vi "Calib_Analyse_fit.vi"(0 "Calib file":path, 1 "Input points":dbl[][](array[numeric]) format="%.2f", 2 "polynomial order":i32=2, 5 "Fixed n":bool=TRUE, 7 "n":dbl=0.45 format="%.2f", 9 "Point selector 3":cluster{"Y":dbl, "X":dbl, "t/f":bool}[](array[cluster]) {"X" format="%.2f"; "Y" format="%.2f"}, 11 "Point selector 4":T1(array[cluster])=[{"Y"=3.5155385742, "Y2"=3.2773117676, "X"=-15.0, "t/f"=FALSE}, {"Y"=3.4946367187, "Y2"=3.3075422363, "X"=-10.0, "t/f"=FALSE}, {"Y"=3.473232666, "Y2"=3.3353713379, "X"=-5.0, "t/f"=FALSE}, {"Y"=3.454592041, "Y2"=3.3658986816, "X"=0.0, "t/f"=FALSE}, {"Y"=3.4246572266, "Y2"=3.3874455566, "X"=5.0, "t/f"=FALSE}, {"Y"=3.398965332, "Y2"=3.4137351074, "X"=10.0, "t/f"=FALSE}, {"Y"=3.362712646484375, "Y2"=3.428485595703125, "X"=15.0, "t/f"=FALSE}] {"Y2" format="%.2f"; "X" format="%.2f"; "Y" format="%.2f"}) -> (4 "Calib const":string[][](array[string])=[["n", "0.405000"], ["A", "7.730378"], ["B", "6.204067"], ["Av % err", "0.204301"]], 6 "Calibration plot":cluster{cluster{dbl, dbl}[]}[](graph)=[{[{0.8450215822560672, 12.972948762710196}, {0.9063644870167936, 13.35352428024258}, {1.0129933166229186, 14.015056729178777}, {1.0924501688964157, 14.50801239851709}, {1.2215481063301497, 15.308944707524116}, {1.3521910897315237, 16.119462585897956}, {1.4772434835777744, 16.895296069694275}]}, {[{0.8450215822560672, 12.97084622363197}, {0.9063644870167936, 13.353228276297402}, {1.0129933166229186, 14.026771757587431}, {1.0924501688964157, 14.499243467101884}, {1.2215481063301497, 15.307992219000921}, {1.3521910897315237, 16.116882250583185}, {1.4772434835777744, 16.898281339562185}]}], 8 "Average Temp":dbl=19.0 format="%.2f", 10 "Point selector 3 out":cluster{"Y":dbl, "X":dbl, "t/f":bool}[](array[cluster]) {"X" format="%.2f"; "Y" format="%.2f"}, 14 "Coefficients":dbl[][](array[numeric]) format="%.2f", 15 "Point selector 4 out":T1(array[cluster])=[{"Y"=3.5155385742, "Y2"=3.2773117676, "X"=-15.0, "t/f"=FALSE}, {"Y"=3.4946367187, "Y2"=3.3075422363, "X"=-10.0, "t/f"=FALSE}, {"Y"=3.473232666, "Y2"=3.3353713379, "X"=-5.0, "t/f"=FALSE}, {"Y"=3.454592041, "Y2"=3.3658986816, "X"=0.0, "t/f"=FALSE}, {"Y"=3.4246572266, "Y2"=3.3874455566, "X"=5.0, "t/f"=FALSE}, {"Y"=3.398965332, "Y2"=3.4137351074, "X"=10.0, "t/f"=FALSE}, {"Y"=3.362712646484375, "Y2"=3.428485595703125, "X"=15.0, "t/f"=FALSE}] {"Y2" format="%.2f"; "X" format="%.2f"; "Y" format="%.2f"})   [LabVIEW 2022 SP3]
uses:
  <vilib>/Analysis/baseanly.llb/Mean (DBL).vi
  Globals/Calib_global.vi
  Acquisition/PWA/PWAtasksGLOBAL.vi
  <vilib>/Analysis/NI_AALBase.lvlib
panel:
  out "GMU:Source:ppm/%Density":dbl format="%.2f"
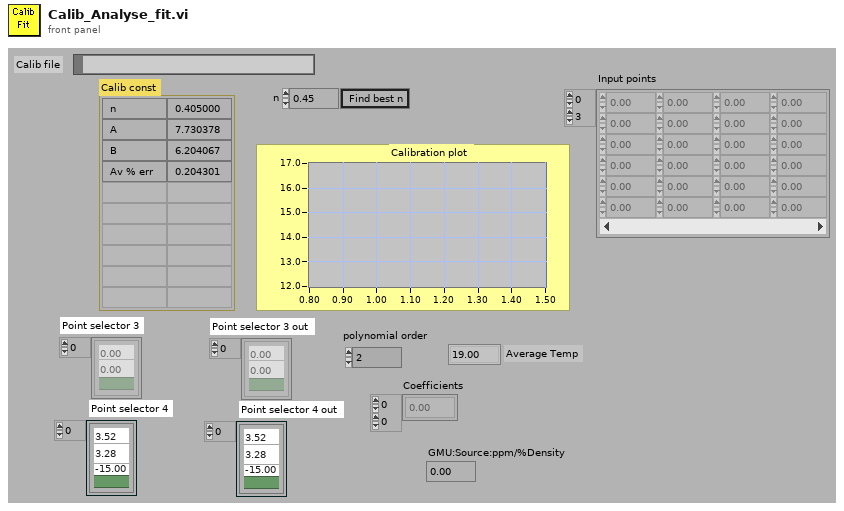
[diagram p1: front panel]
types:
  T1 = cluster{"Y":dbl, "Y2":dbl, "X":dbl, "t/f":bool}[]
  T2 = typedef "Cal_Inst_type.ctl" = enum16{"Propeller anemometer", "Pressure Transducer", "Hot wire", "Cross wire velocity", "Cross wire angle", "Generic Linear", "Generic Polynomial", "Poly Fit Special", "Fast FID", "Thermocouple", "Cold wire", "Pulsed Wire"}
  T3 = cluster{"Y":dbl, "Y":dbl, "X":dbl, "switch":bool}
  T4 = typedef "Ref_Inst_type.ctl" = enum16{"Propellor anemometer", "Pressure Transducer", "Raw voltage", "Pitot-static tube", "Generic Linear", "Generic Polynomial", "Thermocouple", "LDA", "Enter Value", "ADAM Channel"}
  T5 = typedef "zeroableInst.ctl" = enum32{"Zeroable", "Do Not Zero"}
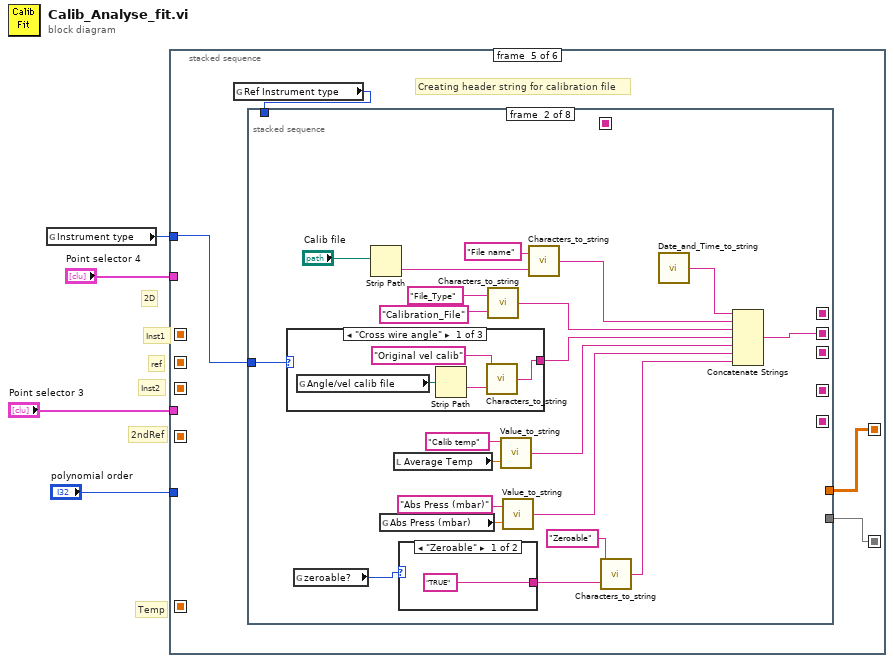
[diagram p0: block diagram]
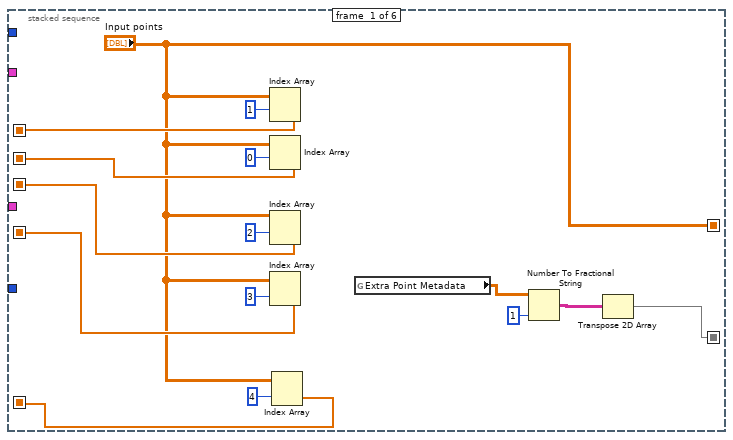
[diagram p2: hidden frame]
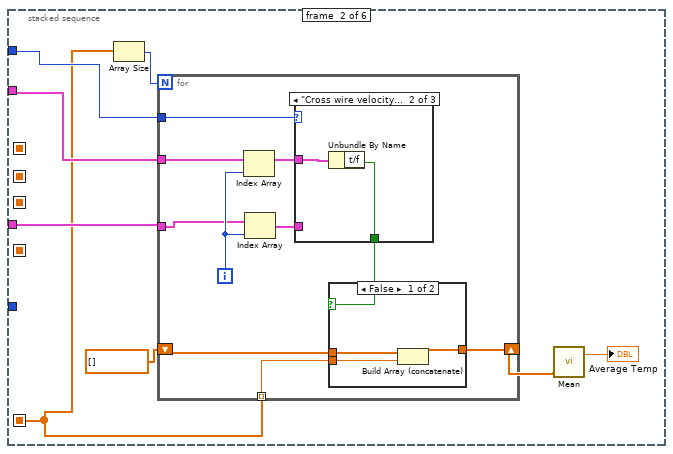
[diagram p3: hidden frame]
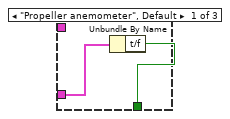
[diagram p5: hidden frame]
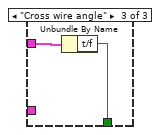
[diagram p6: hidden frame]
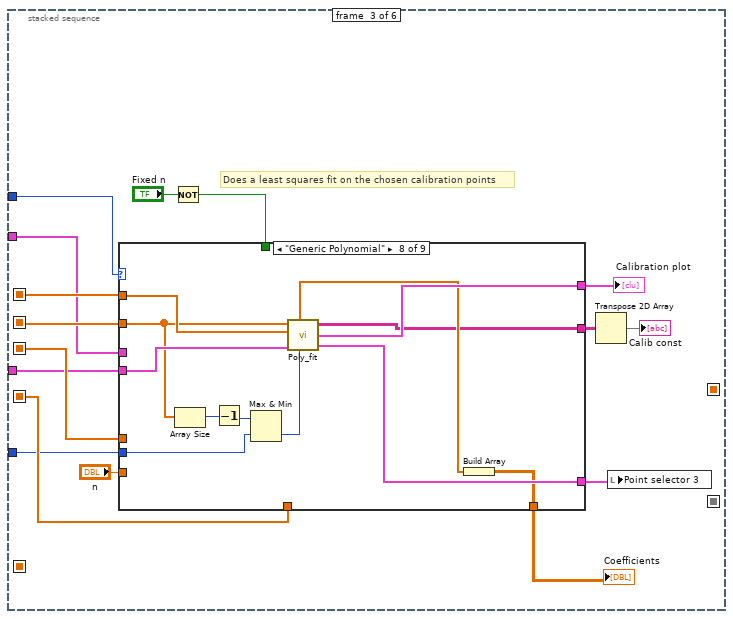
[diagram p7: hidden frame]
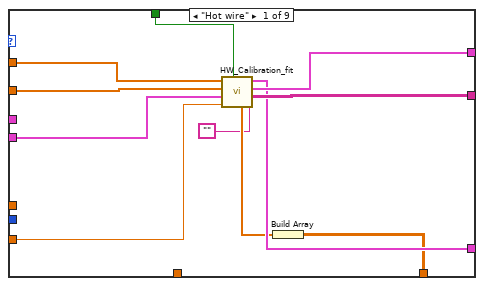
[diagram p8: hidden frame]
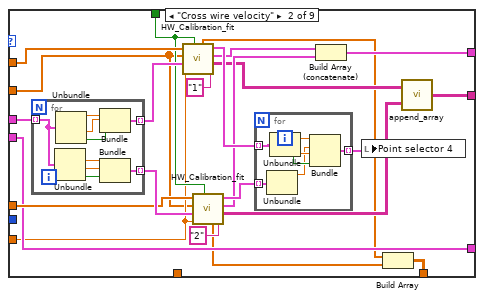
[diagram p9: hidden frame]
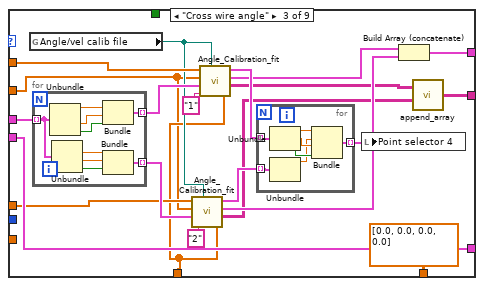
[diagram p10: hidden frame]
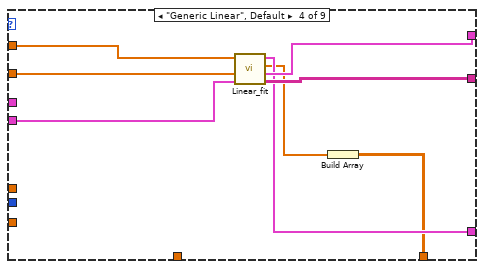
[diagram p11: hidden frame]
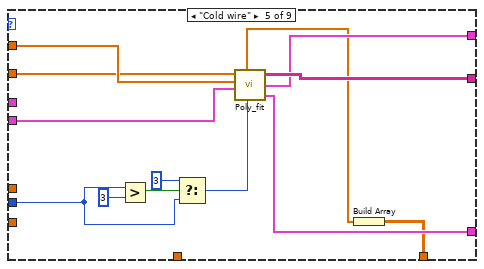
[diagram p12: hidden frame]
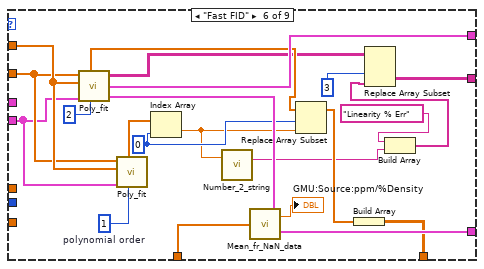
[diagram p13: hidden frame]
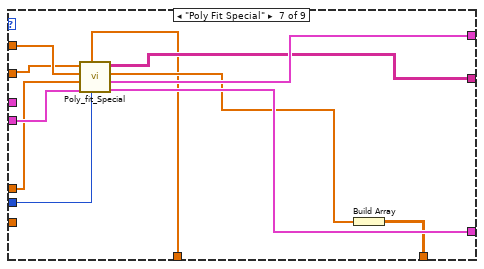
[diagram p14: hidden frame]
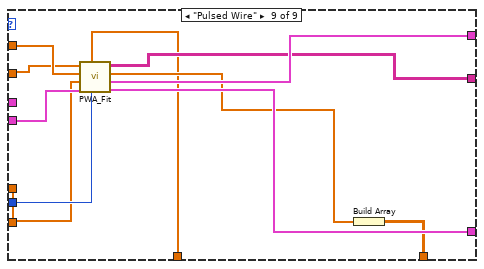
[diagram p15: hidden frame]
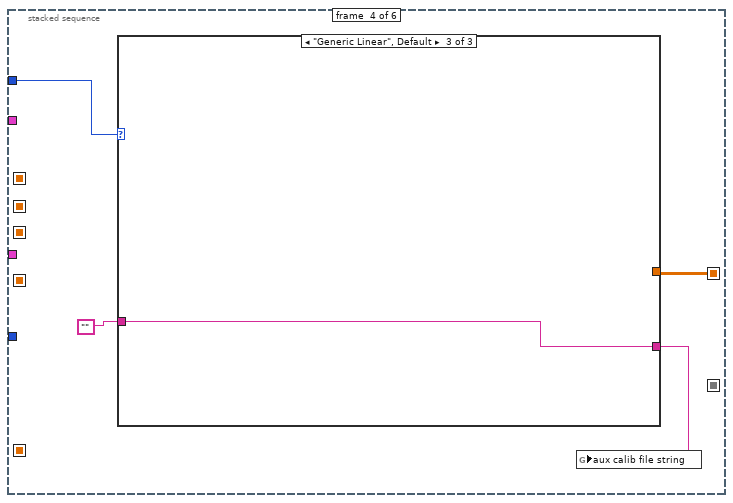
[diagram p16: hidden frame]
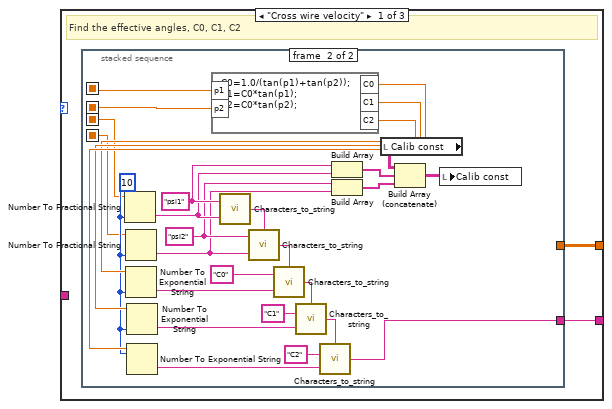
[diagram p17: hidden frame]
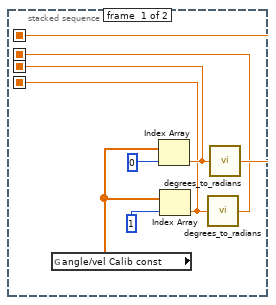
[diagram p18: hidden frame]
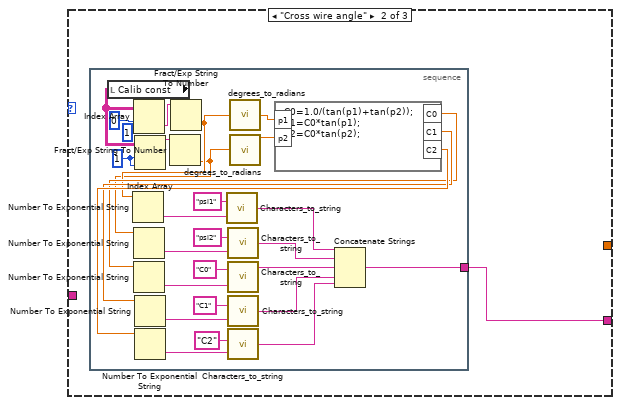
[diagram p19: hidden frame]
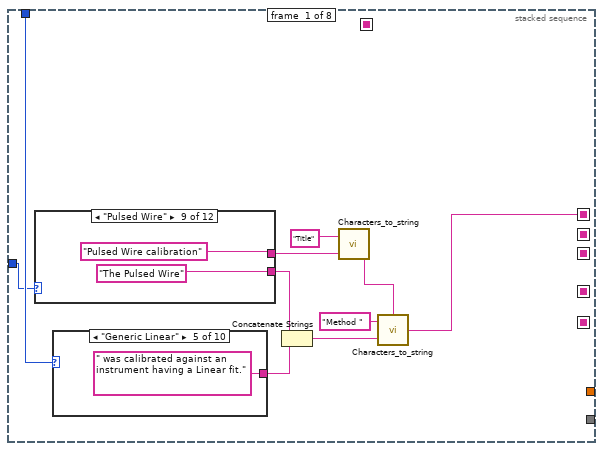
[diagram p20: hidden frame]
diagram:
  # "Temp"
  # "2D"
  # "2ndRef"
  # "Inst2"
  # "Inst1"
  # "ref"
  n1 = global read "Calib_global.vi" "Instrument type"() -> (w4:T2)
  n2 = stacked-sequence {
    seq-local: ["Input points" _ _ _ _ _] -> [_ _ _ w228 w300 _]
    seq-local: [w15 _ _ _ _ _] -> [_ _ w56 _ _ _]
    seq-local: [w14 _ _ _ _ _] -> [_ _ w55 _ _ _]
    seq-local: [w13 _ _ _ _ _] -> [_ _ w54 _ _ _]
    seq-local: [w12 _ _ _ _ _] -> [_ _ w53 _ _ _]
    seq-local: [w9 _ _ _ _ _] -> [_ w21 _ _ _ _]
    seq-local: [w5 _ _ _ _ _] -> [_ _ _ _ w298 _]
    tunnel: w4 -> [_ w27 w50 w227 w299 _]
    tunnel: "Point selector 3" -> [_ w26 w52 _ _ _]
    tunnel: "Point selector 4" -> [_ w25 w51 _ _ _]
    tunnel: "polynomial order" -> [_ _ w48 _ _ _]
    frame #0 {
      n3 = Index Array(array="Input points", index (row)=1) -> (element=w15:dbl[])  [unwired: 1 in]
      n4 = Index Array(array="Input points", index (row)=0) -> (element=w14:dbl[])  [unwired: 1 in]
      n5 = Index Array(array="Input points", index (row)=2) -> (element=w13:dbl[])  [unwired: 1 in]
      n6 = Index Array(array="Input points", index (row)=3) -> (element=w12:dbl[])  [unwired: 1 in]
      n7 = Index Array(array="Input points", index (row)=4) -> (element=w9:dbl[])  [unwired: 1 in]
      n8 = global read "Calib_global.vi" "Extra Point Metadata"() -> (w8:dbl[][])
      n9 = Number To Fractional String(number=w8, precision (6)=i16 1) -> (F-format string=w6:string[][])  [unwired: 2 in]
      n10 = Transpose 2D Array(2D array=w6) -> (transposed array=w5:string[][])
    }
    frame #1 {
      n11 = Array Size(array=w21) -> (size(s)=w20:i32)
      n12 = for {
        N: w20 -> [_]
        tunnel: w27 -> [w37]
        tunnel: w26 -> [w29]
        tunnel: w25 -> [w31]
        shift-right: [w34] -> w22
        shift-left: dbl[] [] -> [w35]
        tunnel: w21 -> [w33] mode=indexing
        i -> [w30]
        n13 = Index Array(array=w31, index=w30) -> (element=w32:cluster{"Y":dbl, "Y2":dbl, "X":dbl, "t/f":bool})
        n14 = Index Array(array=w29, index=w30) -> (element=w28:cluster{"Y":dbl, "X":dbl, "t/f":bool})
        n15 = case shown="\"Cross wire velocity\"" w37 {
          tunnel: w28 -> [w43 _ _]
          tunnel: w32 -> [_ w45 w47]
          tunnel: [w42 w44 w46] -> w36
          frame "Propeller anemometer", Default {
            n16 = Unbundle By Name(w43) -> ("t/f"=w42:bool)
          }
          frame "Cross wire velocity" {
            n17 = Unbundle By Name(w45) -> ("t/f"=w44:bool)
          }
          frame "Cross wire angle" {
            n18 = Unbundle By Name(w47) -> ("t/f"=w46:bool)
          }
        }
        n19 = case shown="False" w36 {
          tunnel: w35 -> [w40 w41]
          tunnel: [w39 w41] -> w34
          tunnel: w33 -> [w38 _]
          frame False {
            n20 = Build Array (concatenate)(w40, w38) -> (w39:dbl[])
          }
          frame True {
          }
        }
      }
      n21 = call-poly <vilib>:"Mean.vi"("X"=w22) -> ("mean"=→"Average Temp":dbl)  [unwired: 1 out]
    }
    frame #2 {
      # "Does a least squares fit on the chosen calibration points"
      n22 = Not(x="Fixed n") -> (.not. x?=w58:bool)
      n23 = case shown="\"Generic Polynomial\"" w50 {
        tunnel: [w69 w87 w125 w153 w168 w191 w202 w214 w225] -> w61
        tunnel: w56 -> [w74 w97 w134 w158 w167 w180 w200 w209 w223]
        tunnel: w55 -> [w73 w75 w114 w157 w166 w179 w199 w208 w222]
        tunnel: w58 -> [w72 w85 _ _ _ _ _ _ _]
        tunnel: w51 -> [_ w88 w126 _ _ _ _ _ _]
        tunnel: [w71 w81 w119 w156 w171 w181 w196 w210 w219] -> w59
        tunnel: [w70 w89 w127 w155 w170 w192 w203 w215 w226] -> w60
        tunnel: w54 -> [_ w93 w116 _ _ _ w194 _ w217]
        tunnel: w52 -> [w68 w87 w125 w154 w169 w178 w198 w212 w221]
        tunnel: "n" -> [w67 w84 _ _ _ _ _ _ _]
        tunnel: w53 -> [_ _ w115 _ _ w173 w193 _ w216]
        tunnel: [w65 w78 dbl[][] [[0.0, 0.0], [0.0, 0.0]] w151 w160 w190 w201 w213 w224] -> w49
        tunnel: w48 -> [_ _ _ _ w159 _ w195 w205 w218]
        frame "Hot wire" {
          n24 = call "HW_Calibration_fit.vi"("coeff suffix"="", "Fixed n (F)"=w72, "n input  (0.45)"=w67, "Point selector"=w68, "Velocity"=w73, "HW voltage"=w74) -> ("Calib const"=w71:string[][], "Calibration plot"=w70:cluster{cluster{dbl, "mse":dbl}[]}[], "Point selector"=w69:cluster{"Y":dbl, "X":dbl, "switch":bool}[], "Coefficients"=w66:dbl[])
          n25 = Build Array(w66) -> (w65:dbl[][])
        }
        frame "Cross wire velocity" {
          n26 = for {
            tunnel: w88 -> [w109] mode=indexing
            tunnel: [w110] -> w96 mode=indexing
            tunnel: [w108] -> w94 mode=indexing
            n27 = Unbundle(w109) -> ("Y2"=w107:dbl, "X"=w106:dbl, "t/f"=w105:bool)  [unwired: 1 out]
            n28 = Unbundle(w109) -> ("Y"=w113:dbl, "X"=w112:dbl, "t/f"=w111:bool)  [unwired: 1 out]
            n29 = Bundle("Y"=w113, "X"=w112, "t/f"=w111) -> (w110:cluster{"Y":dbl, "X":dbl, "t/f":bool})  [unwired: 1 out]
            n30 = Bundle("Y2"=w107, "X"=w106, "t/f"=w105) -> (w108:cluster{"Y2":dbl, "X":dbl, "t/f":bool})  [unwired: 1 out]
          }
          n31 = call "HW_Calibration_fit.vi"("coeff suffix"="1", "Fixed n (F)"=w85, "n input  (0.45)"=w84, "Point selector"=w96, "Velocity"=w75, "HW voltage"=w97) -> ("Calib const"=w82:string[][], "Calibration plot"=w90:cluster{cluster{dbl, "mse":dbl}[]}[], "Point selector"=w95:cluster{"Y":dbl, "X":dbl, "switch":bool}[], "Coefficients"=w76:dbl[])
          n32 = call "HW_Calibration_fit.vi"("coeff suffix"="2", "Fixed n (F)"=w85, "n input  (0.45)"=w84, "Point selector"=w94, "Velocity"=w75, "HW voltage"=w93) -> ("Calib const"=w83:string[][], "Calibration plot"=w91:cluster{cluster{dbl, "mse":dbl}[]}[], "Point selector"=w92:cluster{"Y":dbl, "X":dbl, "switch":bool}[], "Coefficients"=w77:dbl[])
          n33 = for {
            tunnel: w95 -> [w104] mode=indexing
            tunnel: [w100] -> w86 mode=indexing
            tunnel: w92 -> [w99] mode=indexing
            n34 = Unbundle(w99) -> ("Y"=w98:dbl)  [unwired: 2 out]
            n35 = Unbundle(w104) -> ("Y"=w103:dbl, "X"=w102:dbl, "switch"=w101:bool)
            n36 = Bundle("Y"=w103, "Y"=w98, "X"=w102, "switch"=w101) -> (w100:T3)  [unwired: 1 out]
          }
          n37 = Build Array (concatenate)(w90, w91) -> (w89:cluster{cluster{dbl, "mse":dbl}[]}[])
          n38 = local write "Point selector 4"(w86) -> ()
          n39 = Build Array(w76, w77) -> (w78:dbl[][])
          n40 = call "append_array.vi"("array 2"=w83, "array 1"=w82) -> ("appended array"=w81:string[][])
        }
        frame "Cross wire angle" {
          n41 = global read "Calib_global.vi" "Angle/vel calib file"() -> (w118:path)
          n42 = for {
            tunnel: w126 -> [w146] mode=indexing
            tunnel: [w147] -> w133 mode=indexing
            tunnel: [w145] -> w131 mode=indexing
            n43 = Unbundle(w146) -> ("Y"=w150:dbl, "X"=w149:dbl, "t/f"=w148:bool)  [unwired: 1 out]
            n44 = Unbundle(w146) -> ("Y2"=w144:dbl, "X"=w143:dbl, "t/f"=w142:bool)  [unwired: 1 out]
            n45 = Bundle("Y"=w150, "X"=w149, "t/f"=w148) -> (w147:cluster{"Y":dbl, "X":dbl, "t/f":bool})  [unwired: 1 out]
            n46 = Bundle("Y2"=w144, "X"=w143, "t/f"=w142) -> (w145:cluster{"Y2":dbl, "X":dbl, "t/f":bool})  [unwired: 1 out]
          }
          n47 = call "Angle_Calibration_fit.vi"("Reference Velocity"=w115, "Vel calib file"=w118, "coeff suffix"="2", "Point selector"=w131, "Angle"=w114, "HW voltage"=w116) -> ("Calib const"=w120:string[][], "Angle calibration (output)"=w129:cluster{cluster{"Y":dbl, "Y":dbl}[]}[], "Point selector"=w130:cluster{"Y":dbl, "X":dbl, "switch":bool}[])
          n48 = call "Angle_Calibration_fit.vi"("Reference Velocity"=w115, "Vel calib file"=w118, "coeff suffix"="1", "Point selector"=w133, "Angle"=w114, "HW voltage"=w134) -> ("Calib const"=w121:string[][], "Angle calibration (output)"=w128:cluster{cluster{"Y":dbl, "Y":dbl}[]}[], "Point selector"=w132:cluster{"Y":dbl, "X":dbl, "switch":bool}[])
          n49 = for {
            tunnel: w132 -> [w141] mode=indexing
            tunnel: [w137] -> w124 mode=indexing
            tunnel: w130 -> [w136] mode=indexing
            n50 = Unbundle(w141) -> ("Y"=w140:dbl, "X"=w139:dbl, "switch"=w138:bool)
            n51 = Unbundle(w136) -> ("Y"=w135:dbl)  [unwired: 2 out]
            n52 = Bundle("Y"=w140, "Y"=w135, "X"=w139, "switch"=w138) -> (w137:T3)  [unwired: 1 out]
          }
          n53 = local write "Point selector 4"(w124) -> ()
          n54 = Build Array (concatenate)(w128, w129) -> (w127:cluster{cluster{"Y":dbl, "Y":dbl}[]}[])
          n55 = call "append_array.vi"("array 2"=w120, "array 1"=w121) -> ("appended array"=w119:string[][])
        }
        frame "Generic Linear", Default {
          n56 = call "Linear_fit.vi"("Point selector"=w154, "Input X array"=w157, "Input Y array"=w158) -> ("Calib const"=w156:string[][], "Calibration plot"=w155:cluster{cluster{dbl, dbl}[]}[], "Coefficients"=w152:dbl[], "Point selector"=w153:cluster{"Y":dbl, "X":dbl, "switch":bool}[])  [unwired: 1 out]
          n57 = Build Array(w152) -> (w151:dbl[][])
        }
        frame "Cold wire" {
          n58 = Greater?(x=w159, y=3) -> (0:w164:bool)
          n59 = Select(t=3, s=w164, f=w159) -> (s? t:f=w162:i32)
          n60 = call "Poly_fit.vi"("Input Y array"=w166, "Input X array"=w167, "polynomial order"=w162, "Point selector"=w169) -> ("Coefficients"=w161:dbl[], "Calib const"=w171:string[][], "Calibration plot"=w170:cluster{cluster{dbl, dbl}[]}[], "Point selector"=w168:cluster{"Y":dbl, "X":dbl, "switch":bool}[])  [unwired: 1 out]
          n61 = Build Array(w161) -> (w160:dbl[][])
        }
        frame "Fast FID" {
          w185 = 0 ("index")
          w188 = 1  # polynomial order
          n62 = call "Poly_fit.vi"("Input Y array"=w179, "Input X array"=w180, "polynomial order"=2, "Point selector"=w178) -> ("Coefficients"=w186:dbl[], "Calib const"=w183:string[][], "Calibration plot"=w192:cluster{cluster{dbl, dbl}[]}[], "Point selector"=w191:cluster{"Y":dbl, "X":dbl, "switch":bool}[])  [unwired: 1 out]
          n63 = call "Poly_fit.vi"("Input Y array"=w179, "Input X array"=w180, "polynomial order"=w188, "Point selector"=w178) -> ("Coefficients"=w187:dbl[])  [unwired: 4 out]
          n64 = Index Array(array=w187, index=w185) -> (element=w177:dbl)
          n65 = call "Number_2_string.vi"("number"=w177) -> ("String"=w175:string)  [unwired: 1 in]
          n66 = call "Mean_fr_NaN_data.vi"("Data"=w173) -> ("Mean value"=→"GMU:Source:ppm/%Density":dbl)  [unwired: 1 out]
          n67 = Replace Array Subset(array=w186, new element=w177, index=w185) -> (w184:dbl[])
          n68 = Build Array(w184) -> (w190:dbl[][])
          n69 = Build Array("Linearity % Err" ("new element/subarray"), w175) -> (w174:string[])
          n70 = Replace Array Subset(array=w183, new element=w174, index (col)=3 ("disabled index (col)")) -> (w181:string[][])  [unwired: 1 in]
        }
        frame "Poly Fit Special" {
          n71 = call "Poly_fit_Special.vi"("polynomial order"=w195, "Input X^3"=w193, "Point selector"=w198, "Input X^2"=w194, "Input X array"=w200, "Input Y array"=w199) -> ("Point selector"=w202:cluster{"Y":dbl, "X":dbl, "switch":bool}[], "Calibration plot"=w203:cluster{cluster{dbl, dbl}[]}[], "Coefficients"=w197:dbl[], "Calib const"=w196:string[][])
          n72 = Build Array(w197) -> (w201:dbl[][])
        }
        frame "Generic Polynomial" {
          n73 = Array Size(array=w208) -> (size(s)=w207:i32)
          n74 = Decrement(x=w207) -> (x-1=w206:i32)
          n75 = Max & Min(x=w206, y=w205) -> (min(x,y)=w204:i32)  [unwired: 1 out]
          n76 = call "Poly_fit.vi"("Input Y array"=w208, "Input X array"=w209, "polynomial order"=w204, "Point selector"=w212) -> ("Coefficients"=w211:dbl[], "Calib const"=w210:string[][], "Calibration plot"=w215:cluster{cluster{dbl, dbl}[]}[], "Point selector"=w214:cluster{"Y":dbl, "X":dbl, "switch":bool}[])  [unwired: 1 out]
          n77 = Build Array(w211) -> (w213:dbl[][])
        }
        frame "Pulsed Wire" {
          n78 = call "PWA_Fit.vi"("polynomial order"=w218, "Input X^3"=w216, "Point selector"=w221, "Input X^2"=w217, "Input X array"=w223, "Input Y array"=w222) -> ("Point selector"=w225:cluster{"Y":dbl, "X":dbl, "switch":bool}[], "Calibration plot"=w226:cluster{cluster{dbl, dbl}[]}[], "Coefficients"=w220:dbl[], "Calib const"=w219:string[][])
          n79 = Build Array(w220) -> (w224:dbl[][])
        }
      }
      "Calibration plot" <- w60
      "Coefficients" <- w49
      n80 = Transpose 2D Array(2D array=w59) -> (transposed array=→"Calib const":string[][])
      n81 = local write "Point selector 3"(w61) -> ()
    }
    frame #3 {
      n82 = case shown="\"Generic Linear\", Default" w227 {
        tunnel: "" -> [_ _ w297]
        tunnel: [w232 w267 w297] -> w230
        tunnel: w228 -> [w231 _ _]
        frame "Cross wire velocity" {
          # "Find the effective angles, C0, C1, C2"
          n83 = stacked-sequence {
            seq-local: [w237 _] -> [_ w248]
            seq-local: [w236 _] -> [_ w246]
            seq-local: [w235 _] -> [_ w247]
            seq-local: [w234 _] -> [_ w245]
            tunnel: [_ w240] -> w232
            tunnel: w231 -> [_ _]
            frame #0 {
              n84 = global read "Calib_global.vi" "angle/vel Calib const"() -> (w233:dbl[])
              n85 = Index Array(array=w233, index=0) -> (element=w235:dbl)
              n86 = Index Array(array=w233, index=1) -> (element=w234:dbl)
              n87 = call "degrees_to_radians.vi"("degrees"=w234) -> ("radians"=w236:dbl)
              n88 = call "degrees_to_radians.vi"("degrees"=w235) -> ("radians"=w237:dbl)
            }
            frame #1 {
              w249 = 10
              w255 = "psi2"
              w257 = "psi1"
              n89 = Number To Fractional String(number=w247, precision (6)=w249) -> (F-format string=w256:string)  [unwired: 2 out]
              n90 = Number To Fractional String(number=w245, precision (6)=w249) -> (F-format string=w254:string)  [unwired: 2 out]
              n91 = formula code="C0=1.0/(tan(p1)+tan(p2));\nC1=C0*tan(p1);\nC2=C0*tan(p2);"("p1"=w248, "p2"=w246) -> ("C0"=w264:dbl, "C1"=w265:dbl, "C2"=w266:dbl)
              n92 = Number To Exponential String(number=w264, precision (6)=w249) -> (E-format string=w262:string)  [unwired: 2 out]
              n93 = Number To Exponential String(number=w265, precision (6)=w249) -> (E-format string=w260:string)  [unwired: 2 out]
              n94 = Number To Exponential String(number=w266, precision (6)=w249) -> (E-format string=w258:string)  [unwired: 2 out]
              n95 = call "Characters_to_string.vi"("Characters to write"=w256, "Label for characters"=w257) -> ("Output string"=w244:string)  [unwired: 1 in]
              n96 = call "Characters_to_string.vi"("stringIn"=w244, "Characters to write"=w254, "Label for characters"=w255) -> ("Output string"=w243:string)
              n97 = call "Characters_to_string.vi"("stringIn"=w243, "Characters to write"=w262, "Label for characters"="C0") -> ("Output string"=w242:string)
              n98 = call "Characters_to_string.vi"("stringIn"=w242, "Characters to write"=w260, "Label for characters"="C1") -> ("Output string"=w241:string)
              n99 = call "Characters_to_string.vi"("stringIn"=w241, "Characters to write"=w258, "Label for characters"="C2") -> ("Output string"=w240:string)
              n100 = Build Array(w257, w256) -> (w253:string[])
              n101 = Build Array(w255, w254) -> (w252:string[])
              n102 = local read "Calib const"() -> (w251:string[][])
              n103 = Build Array (concatenate)(w251, w253, w252) -> (w250:string[][])
              n104 = local write "Calib const"(w250) -> ()
            }
          }
        }
        frame "Cross wire angle" {
          n105 = stacked-sequence {
            tunnel: [w278] -> w267
            frame #0 {
              w277 = 1
              n106 = local read "Calib const"() -> (w275:string[][])
              n107 = Index Array(array=w275, index (row)=0, index (col)=1) -> (element=w274:string)
              n108 = Index Array(array=w275, index (row)=w277, index (col)=w277) -> (element=w273:string)
              n109 = Fract/Exp String To Number(string=w273) -> (number=w268:dbl)  [unwired: 4 out]
              n110 = Number To Exponential String(number=w268) -> (E-format string=w290:string)  [unwired: 3 out]
              n111 = Fract/Exp String To Number(string=w274) -> (number=w271:dbl)  [unwired: 4 out]
              n112 = Number To Exponential String(number=w271) -> (E-format string=w291:string)  [unwired: 3 out]
              n113 = call "Characters_to_string.vi"("Characters to write"=w291, "Label for characters"="psi1") -> ("Output string"=w282:string)  [unwired: 1 in]
              n114 = call "Characters_to_string.vi"("Characters to write"=w290, "Label for characters"="psi2") -> ("Output string"=w281:string)  [unwired: 1 in]
              n115 = call "degrees_to_radians.vi"("degrees"=w271) -> ("radians"=w270:dbl)
              n116 = call "degrees_to_radians.vi"("degrees"=w268) -> ("radians"=w269:dbl)
              n117 = formula code="C0=1.0/(tan(p1)+tan(p2));\nC1=C0*tan(p1);\nC2=C0*tan(p2);"("p1"=w270, "p2"=w269) -> ("C0"=w294:dbl, "C1"=w295:dbl, "C2"=w296:dbl)
              n118 = Number To Exponential String(number=w294) -> (E-format string=w288:string)  [unwired: 3 out]
              n119 = Number To Exponential String(number=w295) -> (E-format string=w286:string)  [unwired: 3 out]
              n120 = Number To Exponential String(number=w296) -> (E-format string=w284:string)  [unwired: 3 out]
              n121 = call "Characters_to_string.vi"("Characters to write"=w288, "Label for characters"="C0") -> ("Output string"=w283:string)  [unwired: 1 in]
              n122 = call "Characters_to_string.vi"("Characters to write"=w286, "Label for characters"="C1") -> ("Output string"=w280:string)  [unwired: 1 in]
              n123 = call "Characters_to_string.vi"("Characters to write"=w284, "Label for characters"="C2") -> ("Output string"=w279:string)  [unwired: 1 in]
              n124 = Concatenate Strings(w282, w281, w283, w280, w279) -> (w278:string)
            }
          }
        }
        frame "Generic Linear", Default {
        }
      }
      n125 = global write "Calib_global.vi" "aux calib file string"(w230) -> ()
    }
    frame #4 {
      # "Creating header string for calibration file"
      n126 = global read "Calib_global.vi" "Ref Instrument type"() -> (w301:T4)
      n127 = stacked-sequence {
        seq-local: [_ w364 _ _ _ _ _ _] -> [_ _ _ _ _ _ _ w686]
        seq-local: [w302 _ _ _ _ _ _ _] -> [_ _ _ _ _ _ _ w687]
        seq-local: [_ _ w378 _ _ _ _ _] -> [_ _ _ _ _ _ _ w685]
        seq-local: [_ _ _ w392 _ _ _ _] -> [_ _ _ _ _ _ _ w682]
        seq-local: [_ _ _ _ _ _ w665 _] -> [_ _ _ _ _ _ _ w683]
        seq-local: [_ _ _ _ _ w499 _ _] -> [_ _ _ _ _ _ w666 _]
        tunnel: w301 -> [w306 _ _ _ _ _ _ _]
        tunnel: w300 -> [_ _ _ _ _ w496 _ _]
        tunnel: w299 -> [w304 w357 _ w390 _ w490 w664 w688]
        tunnel: w298 -> [_ _ _ _ _ w488 _ _]
        frame #0 {
          n128 = case shown="\"Pulsed Wire\"" w304 {
            tunnel: ["Propeller Anemometer velocity calibration" "Pressure Transducer calibration" "Hot wire velocity calibration" "Cross wire velocity calibration" "Cross wire angle calibration" "Fast FID calibration" "Generic Linear calibration" "Generic Polynomial calibration" "Pulsed Wire calibration" "Generic Backwards Polynomial calibration" "Thermocouple calibration" "Cold wire calibration"] -> w310
            tunnel: ["The Propeller Anemometer" "The Pressure Transducer" "The Hot wire" "The Cross wire" "The Cross wire" "The Fast FID" "The Generic Linear Instrument" "The Generic Polynomial Instrument" "The Pulsed Wire" "The Generic Backwards Polynomial Instrument" "The Thermocouple" "The Cold wire"] -> w307
            frame "Propeller anemometer" {
            }
            frame "Pressure Transducer" {
            }
            frame "Hot wire" {
            }
            frame "Cross wire velocity" {
            }
            frame "Cross wire angle" {
            }
            frame "Fast FID" {
            }
            frame "Generic Linear" {
            }
            frame "Generic Polynomial" {
            }
            frame "Pulsed Wire" {
            }
            frame "Poly Fit Special" {
            }
            frame "Thermocouple" {
            }
            frame "Cold wire" {
            }
          }
          n129 = case shown="\"Generic Linear\"" w306 {
            tunnel: [" was calibrated for velocity against a Propeller Anemometer." " was calibrated for pressure against a Pressure Transducer." " was calibrated against a voltage" " was calibrated for velocity against a Pitot-static tube." " was calibrated against an instrument having a Linear fit." " was calibrated against an instrument having a polynomial fit." " was calibrated for temperature against a thermocouple." " was calibrated for velocity against the LDA." " was calibrated against the reading entered by the user." " was calibrated against an ADAM channel."] -> w308
            frame "Propellor anemometer" {
            }
            frame "Pressure Transducer" {
            }
            frame "Raw voltage" {
            }
            frame "Pitot-static tube" {
            }
            frame "Generic Linear" {
            }
            frame "Generic Polynomial" {
            }
            frame "Thermocouple" {
            }
            frame "LDA" {
            }
            frame "Enter Value" {
            }
            frame "ADAM Channel" {
            }
          }
          n130 = Concatenate Strings(w307, w308) -> (w305:string)
          n131 = call "Characters_to_string.vi"("Characters to write"=w310, "Label for characters"="Title") -> ("Output string"=w303:string)  [unwired: 1 in]
          n132 = call "Characters_to_string.vi"("stringIn"=w303, "Characters to write"=w305, "Label for characters"="Method ") -> ("Output string"=w302:string)
        }
        frame #1 {
          n133 = case shown="\"Cross wire angle\"" w357 {
            tunnel: [w371 "" w376] -> w360
            frame "Cross wire angle" {
              n134 = global read "Calib_global.vi" "Angle/vel calib file"() -> (w370:path)
              n135 = Strip Path(path=w370) -> (name=w369:string)  [unwired: 1 out]
              n136 = call "Characters_to_string.vi"("Characters to write"=w369, "Label for characters"="Original vel calib") -> ("Output string"=w371:string)  [unwired: 1 in]
            }
            frame "Generic Linear", Default {
            }
            frame "Fast FID" {
              n137 = local read "GMU:Source:ppm/%Density"() -> (w375:dbl)
              n138 = call "Value_to_string.vi"("Value"=w375, "Label for value"="GMU:Source:ppm/%Density") -> ("Output string"=w376:string)  [unwired: 1 in]
            }
          }
          n139 = global read "Calib_global.vi" "zeroable?"() -> (w347:T5)
          n140 = Strip Path(path="Calib file") -> (name=w354:string)  [unwired: 1 out]
          n141 = global read "Calib_global.vi" "Abs Press (mbar)"() -> (w359:dbl)
          n142 = local read "Average Temp"() -> (w356:dbl)
          n143 = case shown="\"Zeroable\"" w347 {
            tunnel: ["TRUE" "FALSE"] -> w349
            frame "Zeroable" {
            }
            frame "Do Not Zero" {
            }
          }
          n144 = call "Characters_to_string.vi"("Characters to write"="Calibration_File", "Label for characters"="File_Type") -> ("Output string"=w350:string)  [unwired: 1 in]
          n145 = call "Value_to_string.vi"("Value"=w356, "Label for value"="Calib temp") -> ("Output string"=w361:string)  [unwired: 1 in]
          n146 = call "Value_to_string.vi"("Value"=w359, "Label for value"="Abs Press (mbar)") -> ("Output string"=w362:string)  [unwired: 1 in]
          n147 = call "Characters_to_string.vi"("Characters to write"=w354, "Label for characters"="File name") -> ("Output string"=w351:string)  [unwired: 1 in]
          n148 = call "Characters_to_string.vi"("Characters to write"=w349, "Label for characters"="Zeroable") -> ("Output string"=w346:string)  [unwired: 1 in]
          n149 = call "Date_and_Time_to_string.vi"() -> ("Date and time (spreadsheet)"=w363:string)  [unwired: 4 in, 1 out]
          n150 = Concatenate Strings(w363, w351, w350, w360, w361, w362, w346) -> (w364:string)
        }
        frame #2 {
          n151 = global read "Calib_global.vi" "Ref Inst present"() -> (w377:bool)
          n152 = case shown="True" w377 {
            tunnel: ["" w385] -> w378
            frame False {
            }
            frame True {
              n153 = global read "Calib_global.vi" "Ref Calib file"() -> (w381:path)
              n154 = Strip Path(path=w381) -> (name=w380:string)  [unwired: 1 out]
              n155 = Concatenate Strings("Ref Inst calib file", "\t", w380, "\r\n") -> (w385:string)
            }
          }
        }
        frame #3 {
          n156 = local read "Calib const"() -> (w386:string[][])
          n157 = Index Array(array=w386, index (col)=1) -> (element=w388:string[])  [unwired: 1 in]
          n158 = case shown="\"Cross wire velocity\"" w390 {
            tunnel: [w407 w420 w425 w434 w447 w458 w470 w476 w487] -> w391
            tunnel: w388 -> [_ _ w428 w437 w450 w461 _ _ _]
            tunnel: [2 ("Index") 3 ("Index") 6 ("Index") 9 ("Index") 6 ("Index") 4 ("Index") 3 ("Index") 2 ("Index") 7 ("Index")] -> w389
            tunnel: ["Av % Err" "Linearity % Err" "Av % Err" "Av % err -ve" "Av % Err" "Av % Err" "Av % Err" "Av % Err" "Av % Err"] -> w387
            tunnel: w386 -> [_ _ _ w439 _ _ _ _ _]
            frame "Propeller anemometer", Default {
              n159 = Build Array("Coeff A", "Coeff B") -> (w407:string[])
            }
            frame "Fast FID" {
              n160 = Build Array("Coeff A", "Coeff B", "Coeff C", "Fast FID Bkgnd", "Fast FID Bkgnd Variance", "FFID Bkgnd Volts", "FFID Bkgnd Time", "FFID Bkgnd Filename") -> (w420:string[])
            }
            frame "Generic Polynomial" {
              n161 = Array Size(array=w428) -> (size(s)=w429:i32)
              n162 = Decrement(x=w429) -> (x-1=w427:i32)
              n163 = Build Array("Coeff A", "Coeff B", "Coeff C", "Coeff D", "Coeff E", "Coeff F") -> (w426:string[])
              n164 = Array Subset(array=w426, length=w427) -> (w425:string[])  [unwired: 1 in]
            }
            frame "Pulsed Wire" {
              n165 = Array Size(array=w437) -> (size(s)=w438:i32)
              n166 = Index Array(array=w439, index (col)=0) -> (element=w436:string[])  [unwired: 1 in]
              n167 = Decrement(x=w438) -> (x-1=w435:i32)
              n168 = Array Subset(array=w436, length=w435) -> (w434:string[])  [unwired: 1 in]
            }
            frame "Poly Fit Special" {
              n169 = Array Size(array=w450) -> (size(s)=w451:i32)
              n170 = Decrement(x=w451) -> (x-1=w449:i32)
              n171 = Build Array("Coeff A", "Coeff B", "Coeff C", "Coeff D", "Coeff E", "Coeff F") -> (w448:string[])
              n172 = Array Subset(array=w448, length=w449) -> (w447:string[])  [unwired: 1 in]
            }
            frame "Cold wire" {
              n173 = Array Size(array=w461) -> (size(s)=w462:i32)
              n174 = Decrement(x=w462) -> (x-1=w460:i32)
              n175 = Build Array("Coeff A", "Coeff B", "Coeff C", "Coeff D") -> (w459:string[])
              n176 = Array Subset(array=w459, length=w460) -> (w458:string[])  [unwired: 1 in]
            }
            frame "Hot wire" {
              n177 = Build Array("Coeff n", "Coeff A", "Coeff B") -> (w470:string[])
            }
            frame "Cross wire angle" {
              n178 = Build Array("psi1", "psi2") -> (w476:string[])
            }
            frame "Cross wire velocity" {
              n179 = Build Array("Coeff n1", "Coeff A1", "Coeff B1", "Av % Err", "Coeff n2", "Coeff A2", "Coeff B2") -> (w487:string[])
            }
          }
          n180 = for {
            shift-right: [w403] -> w395
            shift-left: "\r\n" -> [w404]
            tunnel: w391 -> [w402] mode=indexing
            tunnel: w388 -> [w400]
            i -> [w401]
            n181 = Index Array(array=w400, index=w401) -> (element=w399:string)
            n182 = call "Characters_to_string.vi"("Characters to write"=w399, "Label for characters"=w402) -> ("Output string"=w398:string)  [unwired: 1 in]
            n183 = Concatenate Strings(w404, w398) -> (w403:string)
          }
          n184 = Index Array(array=w388, index=w389) -> (element=w394:string)
          n185 = call "Characters_to_string.vi"("Characters to write"=w394, "Label for characters"=w387) -> ("Output string"=w396:string)  [unwired: 1 in]
          n186 = Concatenate Strings(w395, w396) -> (w392:string)
        }
        frame #4 {
        }
        frame #5 {
          n187 = local read "Point selector 4"() -> (w497:T1)
          n188 = local read "Point selector 3"() -> (w498:cluster{"Y":dbl, "X":dbl, "t/f":bool}[])
          n189 = case shown="\"Fast FID\"" w490 {
            tunnel: [w505 w517 w529 w544 w558 w569 w585 w600 w611 w630 w644 w656] -> w500
            tunnel: w498 -> [w504 w516 w528 _ _ w568 w584 w599 w610 w629 w643 w655]
            tunnel: w497 -> [_ _ _ w542 w557 _ _ _ _ _ _ _]
            tunnel: [w503 w515 w527 w541 w554 w567 w583 w597 w609 w628 w642 w654] -> w494
            tunnel: "1" -> [w502 w514 w526 w538 w551 w565 w577 w592 w607 w623 w640 w652]
            frame "Propeller anemometer" {
              n190 = for {
                tunnel: w504 -> [w513] mode=indexing
                tunnel: [w511] -> w503 mode=indexing
                tunnel: w502 -> [w509]
                n191 = Unbundle By Name(w513) -> ("t/f"=w512:bool)
                n192 = Select(t="NaN not included", s=w512, f=w509) -> (s? t:f=w511:string)
              }
              n193 = Concatenate Strings("Velocity m/s", "\t", "Voltage") -> (w505:string)
            }
            frame "Pressure Transducer" {
              n194 = for {
                tunnel: w516 -> [w523] mode=indexing
                tunnel: [w524] -> w515 mode=indexing
                tunnel: w514 -> [w521]
                n195 = Unbundle By Name(w523) -> ("t/f"=w525:bool)
                n196 = Select(t="NaN not included", s=w525, f=w521) -> (s? t:f=w524:string)
              }
              n197 = Concatenate Strings("Pressure mmH2O", "\t", "Voltage") -> (w517:string)
            }
            frame "Hot wire" {
              n198 = for {
                tunnel: w528 -> [w537] mode=indexing
                tunnel: [w535] -> w527 mode=indexing
                tunnel: w526 -> [w533]
                n199 = Unbundle By Name(w537) -> ("t/f"=w536:bool)
                n200 = Select(t="NaN not included", s=w536, f=w533) -> (s? t:f=w535:string)
              }
              n201 = Concatenate Strings("Velocity m/s", "\t", "Voltage") -> (w529:string)
            }
            frame "Cross wire velocity" {
              w543 = "\t"
              n202 = for {
                tunnel: w542 -> [w550] mode=indexing
                tunnel: [w549] -> w541 mode=indexing
                tunnel: w538 -> [w546]
                n203 = Unbundle By Name(w550) -> ("t/f"=w548:bool)
                n204 = Select(t="NaN not included", s=w548, f=w546) -> (s? t:f=w549:string)
              }
              n205 = Concatenate Strings("Velocity m/s", w543, "Voltage1", w543, "Voltage2") -> (w544:string)
            }
            frame "Cross wire angle" {
              w552 = "\t"
              n206 = for {
                tunnel: w557 -> [w564] mode=indexing
                tunnel: [w562] -> w554 mode=indexing
                tunnel: w551 -> [w560]
                n207 = Unbundle By Name(w564) -> ("t/f"=w563:bool)
                n208 = Select(t="NaN not included", s=w563, f=w560) -> (s? t:f=w562:string)
              }
              n209 = Concatenate Strings("Angle (degrees)", w552, "Voltage1", w552, "Voltage2", w552, "Ref velocity") -> (w558:string)
            }
            frame "Generic Linear" {
              n210 = global read "Calib_global.vi" "calib units"() -> (w566:string)
              n211 = for {
                tunnel: w568 -> [w576] mode=indexing
                tunnel: [w574] -> w567 mode=indexing
                tunnel: w565 -> [w572]
                n212 = Unbundle By Name(w576) -> ("t/f"=w575:bool)
                n213 = Select(t="NaN not included", s=w575, f=w572) -> (s? t:f=w574:string)
              }
              n214 = Concatenate Strings(w566, "\t", "Voltage") -> (w569:string)
            }
            frame "Generic Polynomial" {
              w581 = "\t"
              n215 = global read "Calib_global.vi" "calib units"() -> (w582:string)
              n216 = for {
                tunnel: w584 -> [w591] mode=indexing
                tunnel: [w589] -> w583 mode=indexing
                tunnel: w577 -> [w587]
                n217 = Unbundle By Name(w591) -> ("t/f"=w590:bool)
                n218 = Select(t="NaN not included", s=w590, f=w587) -> (s? t:f=w589:string)
              }
              n219 = Concatenate Strings(w582, w581, "Volts", w581, "Volts^2", w581, "Volts^3", "Temperature") -> (w585:string)
            }
            frame "Pulsed Wire" {
              w594 = "\t"
              n220 = for {
                tunnel: w599 -> [w606] mode=indexing
                tunnel: [w604] -> w597 mode=indexing
                tunnel: w592 -> [w602]
                n221 = Unbundle By Name(w606) -> ("t/f"=w605:bool)
                n222 = Select(t="NaN not included", s=w605, f=w602) -> (s? t:f=w604:string)
              }
              n223 = Concatenate Strings("Velocity or Tau" ("string"), w594, "1/TOF", w594, "(1/TOF)^2", w594, "(1/TOF)^3", w594, "Temperature") -> (w600:string)
            }
            frame "Poly Fit Special" {
              n224 = global read "Calib_global.vi" "calib units"() -> (w608:string)
              n225 = for {
                tunnel: w610 -> [w618] mode=indexing
                tunnel: [w616] -> w609 mode=indexing
                tunnel: w607 -> [w614]
                n226 = Unbundle By Name(w618) -> ("t/f"=w617:bool)
                n227 = Select(t="NaN not included", s=w617, f=w614) -> (s? t:f=w616:string)
              }
              n228 = Concatenate Strings(w608, "\t", "Voltage") -> (w611:string)
            }
            frame "Fast FID" {
              w620 = "\t"
              n229 = call "Black box desired channels.vi"() -> ("Names"=w621:string[])  [unwired: 4 in, 1 out]
              n230 = for {
                tunnel: w629 -> [w639] mode=indexing
                tunnel: [w637] -> w628 mode=indexing
                tunnel: w623 -> [w635]
                n231 = Unbundle By Name(w639) -> ("t/f"=w638:bool)
                n232 = Select(t="NaN not included", s=w638, f=w635) -> (s? t:f=w637:string)
              }
              n233 = for {
                tunnel: w621 -> [w634] mode=indexing
                tunnel: w620 -> [w633]
                tunnel: [w632] -> w619 mode=concatenating
                n234 = Concatenate Strings(w634, w633) -> (w632:string)
              }
              n235 = Concatenate Strings("Concentration (ppm)" ("Substring"), w620, "Voltage", w620, "Stand dev" ("string"), w620, "ppm/%Density" ("string"), w620, "Temperature" ("string"), w620, "Include Point?" ("string"), w620, w619) -> (w630:string)
            }
            frame "Thermocouple" {
              n236 = for {
                tunnel: w643 -> [w651] mode=indexing
                tunnel: [w649] -> w642 mode=indexing
                tunnel: w640 -> [w647]
                n237 = Unbundle By Name(w651) -> ("t/f"=w650:bool)
                n238 = Select(t="NaN not included", s=w650, f=w647) -> (s? t:f=w649:string)
              }
              n239 = Concatenate Strings("Temperature", "\t", "Voltage") -> (w644:string)
            }
            frame "Cold wire" {
              n240 = for {
                tunnel: w655 -> [w663] mode=indexing
                tunnel: [w661] -> w654 mode=indexing
                tunnel: w652 -> [w659]
                n241 = Unbundle By Name(w663) -> ("t/f"=w662:bool)
                n242 = Select(t="NaN not included", s=w662, f=w659) -> (s? t:f=w661:string)
              }
              n243 = Concatenate Strings("Temperature", "\t", "Voltage") -> (w656:string)
            }
          }
          n244 = Number To Exponential String(number=w496, precision (6)=i16 10) -> (E-format string=w495:string[][])  [unwired: 2 out]
          n245 = Build Array (concatenate)(w495, w494, w488) -> (w493:string[][])
          n246 = Transpose 2D Array(2D array=w493) -> (transposed array=w492:string[][])
          n247 = call "2D_array_to_string.vi"("2D data array"=w492, "Column titles  (separated by tabs)"=w500, "Array title"="Calib points label") -> ("Output string"=w499:string)
        }
        frame #6 {
          n248 = case shown="\"Cross wire angle\"" w664 {
            tunnel: [w672 w679] -> w665
            tunnel: w666 -> [w671 w679]
            frame "Cross wire angle" {
              w670 = "\r\n"
              w676 = "Voltage"
              w677 = "\t"
              n249 = global read "Calib_global.vi" "orig vel calib points"() -> (w667:dbl[][])
              n250 = Concatenate Strings("Velocity (m/s)", w677, w676, w677, w676) -> (w674:string)
              n251 = Number To Exponential String(number=w667, precision (6)=10) -> (E-format string=w669:string[][])  [unwired: 2 out]
              n252 = call "2D_array_to_string.vi"("2D data array"=w669, "Column titles  (separated by tabs)"=w674, "Array title"="Original vel calib points") -> ("Output string"=w673:string)
              n253 = Concatenate Strings(w670, w671, w670, w670, w673) -> (w672:string)
            }
            frame "Generic Linear", Default {
            }
          }
        }
        frame #7 {
          n254 = global read "Calib_global.vi" "aux calib file string"() -> (w689:string)
          n255 = call "Add_label_to_string.vi"("String to write"=w689, "File Label"="Auxiliary constants") -> ("Output string"=w692:string)
          n256 = global read "Calib_global.vi" "Instument setup Info"() -> (w681:string)
          n257 = Concatenate Strings(w687, w686, w685, w681, w682, w683) -> (w684:string)
          n258 = case shown="\"Pulsed Wire\"" w688 {
            tunnel: [w694 w703 w708 w714 w726 w731 w736 w747 w757 w768 w773 w778] -> w690
            tunnel: w692 -> [_ _ _ w713 w721 _ _ _ _ _ _ _]
            tunnel: " calib label" -> [w697 w700 w705 _ _ w728 w733 w744 w754 w765 w770 w775]
            tunnel: w684 -> [w696 w699 w704 w710 w719 w727 w732 w739 w753 w762 w769 w774]
            tunnel: "\r\n" -> [_ _ _ w709 w718 _ _ _ _ _ _ _]
            frame "Propeller anemometer" {
              n259 = Concatenate Strings("Prop", w697) -> (w695:string)
              n260 = call "Add_label_to_string.vi"("String to write"=w696, "File Label"=w695) -> ("Output string"=w694:string)
            }
            frame "Pressure Transducer" {
              n261 = Concatenate Strings("Mano", w700) -> (w701:string)
              n262 = call "Add_label_to_string.vi"("String to write"=w699, "File Label"=w701) -> ("Output string"=w703:string)
            }
            frame "Hot wire" {
              n263 = Concatenate Strings("HW", w705) -> (w707:string)
              n264 = call "Add_label_to_string.vi"("String to write"=w704, "File Label"=w707) -> ("Output string"=w708:string)
            }
            frame "Cross wire velocity" {
              n265 = global read "Calib_global.vi" "Angle/vel calib file string"() -> (w711:string)
              n266 = call "Add_label_to_string.vi"("String to write"=w710, "File Label"="Cross wire velocity calib label") -> ("Output string"=w715:string)
              n267 = call "Add_label_to_string.vi"("String to write"=w711, "File Label"="Cross wire angle calib label") -> ("Output string"=w712:string)
              n268 = Concatenate Strings(w715, w709, w713, w709, w709, w712) -> (w714:string)
            }
            frame "Cross wire angle" {
              n269 = global read "Calib_global.vi" "Angle/vel calib file string"() -> (w720:string)
              n270 = call "Add_label_to_string.vi"("String to write"=w720, "File Label"="Cross wire velocity calib label") -> ("Output string"=w723:string)
              n271 = call "Add_label_to_string.vi"("String to write"=w719, "File Label"="Cross wire angle calib label") -> ("Output string"=w722:string)
              n272 = Concatenate Strings(w723, w718, w721, w718, w718, w722) -> (w726:string)
            }
            frame "Generic Linear" {
              n273 = Concatenate Strings("Generic Inst", w728) -> (w729:string)
              n274 = call "Add_label_to_string.vi"("String to write"=w727, "File Label"=w729) -> ("Output string"=w731:string)
            }
            frame "Generic Polynomial" {
              n275 = Concatenate Strings("Generic Polynomial", w733) -> (w734:string)
              n276 = call "Add_label_to_string.vi"("String to write"=w732, "File Label"=w734) -> ("Output string"=w736:string)
            }
            frame "Pulsed Wire" {
              n277 = global read "PWAtasksGLOBAL.vi" "PWA Lookup Table"() -> (w743:dbl[])
              n278 = for {
                tunnel: w743 -> [w752] mode=indexing
                shift-right: [w748] -> w741
                shift-left: "" -> [w749]
                n279 = Number To Exponential String(number=w752) -> (E-format string=w750:string)  [unwired: 3 out]
                n280 = Concatenate Strings(w749, w750, "\r\n") -> (w748:string)
              }
              n281 = Concatenate Strings("Pulsed wire", w744) -> (w745:string)
              n282 = call "Add_label_to_string.vi"("String to write"=w741, "File Label"="Pulsed_wire_lookup_table") -> ("Output string"=w738:string)
              n283 = Concatenate Strings(w739, w738) -> (w737:string)
              n284 = call "Add_label_to_string.vi"("String to write"=w737, "File Label"=w745) -> ("Output string"=w747:string)
            }
            frame "Poly Fit Special" {
              n285 = Concatenate Strings("Generic BackPoly", w754) -> (w755:string)
              n286 = call "Add_label_to_string.vi"("String to write"=w753, "File Label"=w755) -> ("Output string"=w757:string)
            }
            frame "Fast FID" {
              n287 = Concatenate Strings("Fast FID", w765) -> (w766:string)
              n288 = call "Replace_data_in_setup_string.vi"("New data string"="0.00", "Input string"=w762, "Variable name"="Fast FID Bkgnd") -> ("Appended string"=w759:string)
              n289 = call "Replace_data_in_setup_string.vi"("New data string"="0.00", "Input string"=w759, "Variable name"="Fast FID Bkgnd Variance") -> ("Appended string"=w758:string)
              n290 = call "Add_label_to_string.vi"("String to write"=w758, "File Label"=w766) -> ("Output string"=w768:string)
            }
            frame "Thermocouple" {
              n291 = Concatenate Strings("Thermocouple", w770) -> (w771:string)
              n292 = call "Add_label_to_string.vi"("String to write"=w769, "File Label"=w771) -> ("Output string"=w773:string)
            }
            frame "Cold wire" {
              n293 = Concatenate Strings("Cold wire", w775) -> (w776:string)
              n294 = call "Add_label_to_string.vi"("String to write"=w774, "File Label"=w776) -> ("Output string"=w778:string)
            }
          }
          n295 = global write "Calib_global.vi" "Header string"(w690) -> ()
        }
      }
    }
    frame #5 {
      n296 = local read "Point selector 4"() -> (→"Point selector 4 out":T1)
      n297 = local read "Point selector 3"() -> (→"Point selector 3 out":cluster{"Y":dbl, "X":dbl, "t/f":bool}[])
    }
  }
